vi "Configure923xAcquisition.vi"(8 "error in (no error)":errorcluster) -> (0 "error out":errorcluster, 1 "Register Channel Status Tags":T1[](array[typedef]), 2 "Register Waveform TDMS Properties":T3[](array[typedef]), 3 "923x Acquisition Config":T5={"NumberOfModules"=0, "Dynamic FPGA VI Ref"=refnum, "KeyphasorX3"=[], "FixedSizeX24"={"EnabledChannels"=[], "Sensitivity"=[], "InputConfig"=[]}, "SamplingInfo"={"Number of Channels"=4, "Sampling Rate"=4.0, "Channels"=[], "Units"=[]}, "BlockSize (sec)"=0.0, "Samples To Read (per chan)"=0, "RunningAcquisitionLength"=0.0, "Settling Time"=0.0, "Waveform Groups"=[], "Acquisition Block Number"=0, "Device Name"="", "ValidConfig"=FALSE} {"FixedSizeX24"."InputConfig" items=["AC Coupled", "DC Coupled", "IEPE AC Coupled"]}, 5 "valid":bool)   [LabVIEW 2015]
uses:
  <vilib>/addons/InsightCM/Devices/Shared/AcquireBaseLoop/controls/Configuration.ctl
  <vilib>/addons/InsightCM/Devices/Shared/AcquireBaseLoop/controls/TachometerConfig.ctl
  <vilib>/addons/InsightCM/Devices/Shared/AcquireBaseLoop/controls/FixedSizeArrays.ctl
  <vilib>/LabVIEW Targets/FPGA/cRIO/shared/nicrio_ModuleControls/nicrio_cRIO-9232_ConfigModeRing.ctl
  <vilib>/addons/InsightCM/Devices/Shared/cRIOWfmAcq/subVIs/RIO Wfm Cust Ctrls/rwfm_SamplingInfo.ctl
  <vilib>/addons/InsightCM/Devices/Shared/AcquireBaseLoop/controls/Group.ctl
  <vilib>/addons/InsightCM/Devices/Shared/AcquireBaseLoop/controls/Channel.ctl
  <vilib>/addons/InsightCM/Utilities/ChannelStatus/controls/RangeParams.ctl
  <vilib>/addons/InsightCM/Devices/Shared/TdmsCreator/controls/RegisterWaveformTdmsPropertiesRoutedMessage.ctl
  <vilib>/addons/InsightCM/Devices/Shared/TdmsCreator/controls/Waveform.ctl
  <vilib>/addons/InsightCM/Devices/Shared/TagPublish/controls/PointToPublish.ctl
  <vilib>/addons/PointValueMap/controls/DataTypes.ctl
  <vilib>/addons/InsightCM/Utilities/GlobalConfiguration/GlobalConfiguration.lvlib
  <vilib>/addons/InsightCM/Devices/Shared/AcquireBaseLoop/FpgaAcquisition923x.lvlib
  <vilib>/addons/InsightCM/Devices/Shared/cRIOWfmAcq/cRIOWfmLib.lvlib
  <vilib>/addons/InsightCM/Utilities/ChannelStatus/ChannelStatus.lvlib
  <vilib>/addons/InsightCM/Devices/Shared/TdmsCreator/TdmsCreator.lvlib
  <vilib>/addons/PointValueMap/PointValueMap.lvlib
  <vilib>/addons/InsightCM/Devices/Shared/TagPublish/TagPublish.lvlib
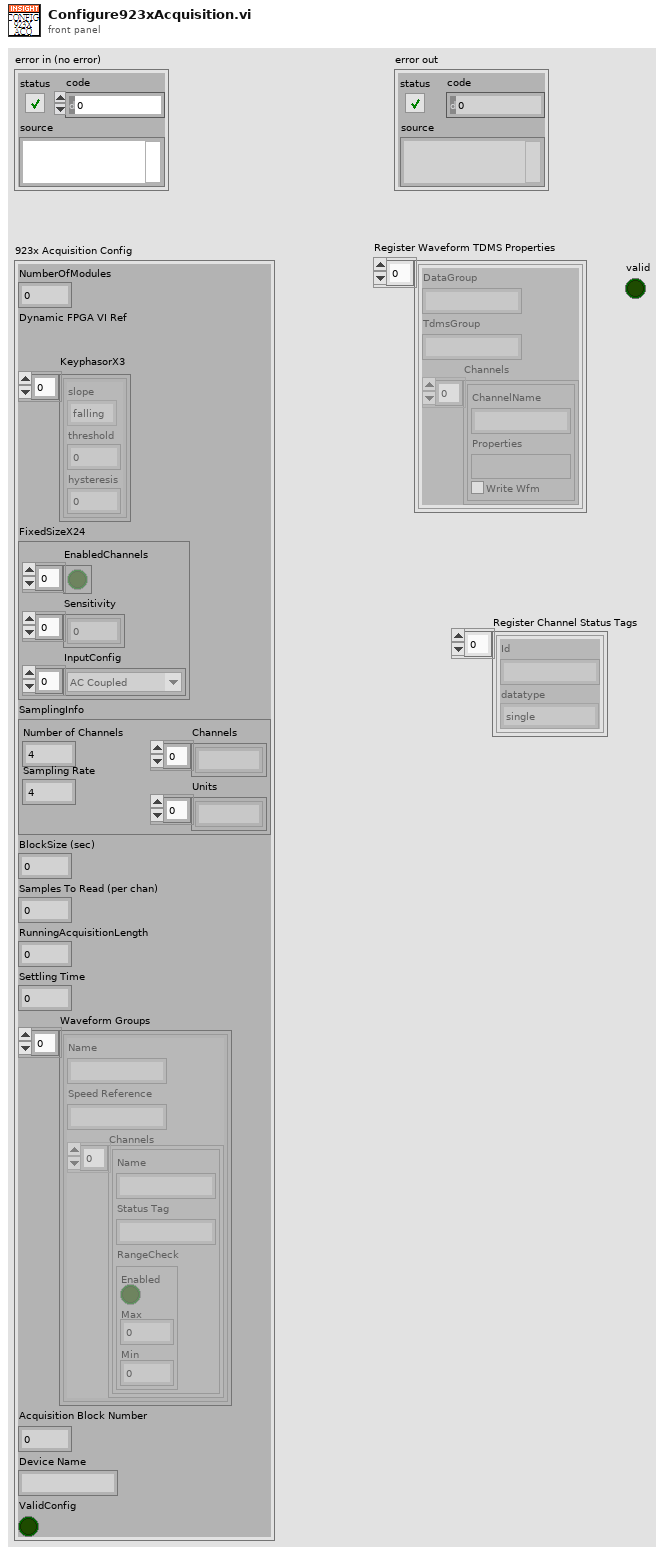
[diagram p1: front panel]
types:
  T1 = typedef "TagPublish.lvlib/PointToPublish.ctl" = cluster{"Id":string, "datatype":T2}
  T2 = typedef "PointValueMap.lvlib/DataTypes.ctl" = enum16{"single", "double", "i32", "string", "variant"}
  T3 = typedef "TdmsCreator.lvlib/RegisterWaveformTdmsPropertiesRoutedMessage.ctl" = cluster{"DataGroup":string, "TdmsGroup":string, "Channels":T4[]}
  T4 = typedef "TdmsCreator.lvlib/Waveform.ctl" = cluster{"ChannelName":string, "Properties":variant, "Write Wfm":bool}
  T5 = typedef "FpgaAcquisition923x.lvlib/Configuration.ctl" = cluster{"NumberOfModules":i16, "Dynamic FPGA VI Ref":refnum<k20>, "KeyphasorX3":T6[], "FixedSizeX24":T7, "SamplingInfo":T9, "BlockSize (sec)":dbl, "Samples To Read (per chan)":i32, "RunningAcquisitionLength":dbl, "Settling Time":dbl, "Waveform Groups":T10[], "Acquisition Block Number":i32, "Device Name":string, "ValidConfig":bool}
  T6 = typedef "FpgaAcquisition923x.lvlib/TachometerConfig.ctl" = cluster{"slope":enum16{"falling", "rising"}, "threshold":dbl, "hysteresis":dbl}
  T7 = typedef "FpgaAcquisition923x.lvlib/FixedSizeArrays.ctl" = cluster{"EnabledChannels":bool[], "Sensitivity":dbl[], "InputConfig":T8[]}
  T8 = typedef "nicrio_cRIO-9232_ConfigModeRing.ctl" = u8
  T9 = typedef "cRIOWfmLib.lvlib/rwfm_SamplingInfo.ctl" = cluster{"Number of Channels":i32, "Sampling Rate":dbl, "Channels":string[], "Units":string[]}
  T10 = typedef "FpgaAcquisition923x.lvlib/Group.ctl" = cluster{"Name":string, "Speed Reference":string, "Channels":T11[]}
  T11 = typedef "FpgaAcquisition923x.lvlib/Channel.ctl" = cluster{"Name":string, "Status Tag":string, "RangeCheck":T12}
  T12 = typedef "ChannelStatus.lvlib/RangeParams.ctl" = cluster{"Enabled":bool, "Max":dbl, "Min":dbl}
  T13 = typedef "Device.ctl" = cluster{"Id":string, "Name":string, "DeviceType":string, "HardwareName":string, "IpAddress":string, "HardwareInfo":T14[], "ApplicationType":string, "ApplicationVersion":string, "EquipmentIds":string[], "ConfigurationVersion":string, "Properties":T14[], "DataGroups":T15[]}
  T14 = typedef "KeyValuePair.ctl" = cluster{"Key":string, "Value":string}
  T15 = typedef "DataGroup.ctl" = cluster{"Name":string, "OperatingStates":T16[], "Properties":T14[], "EquipmentIds":string[]}
  T16 = typedef "OperatingState.ctl" = cluster{"Name":string, "Properties":T14[], "Triggers":T17[]}
  T17 = typedef "Trigger.ctl" = cluster{"Type":string, "Expression":string, "Conditions":T18[]}
  T18 = typedef "Condition.ctl" = cluster{"Source":string, "Type":string, "Operator":string, "CompareTo":string, "DwellSeconds":dbl}
  T19 = typedef "Channel.ctl" = cluster{"Id":string, "DeviceId":string, "Name":string, "ChannelType":string, "HardwareKey":string, "HardwareChannel":string, "DataGroup":string, "Keywords":string[], "EquipmentIds":string[], "Properties":T14[], "Metrics":T20[]}
  T20 = typedef "MetricModel.ctl" = cluster{"Id":string, "MetricDefinitionInstanceId":string, "Properties":T14[]}
  T21 = typedef "Equipment.ctl" = cluster{"Id":string, "ParentId":string, "Levelname":string, "Name":string, "Properties":T14[]}
  T22 = typedef "Tag.ctl" = cluster{"Id":string, "Path":string, "Name":string, "Datatype":string, "Props":T14[], "Keywords":string[]}
  T23 = typedef "SectionKeyValues.ctl" = cluster{"Section":string, "KeyValues":T14[]}
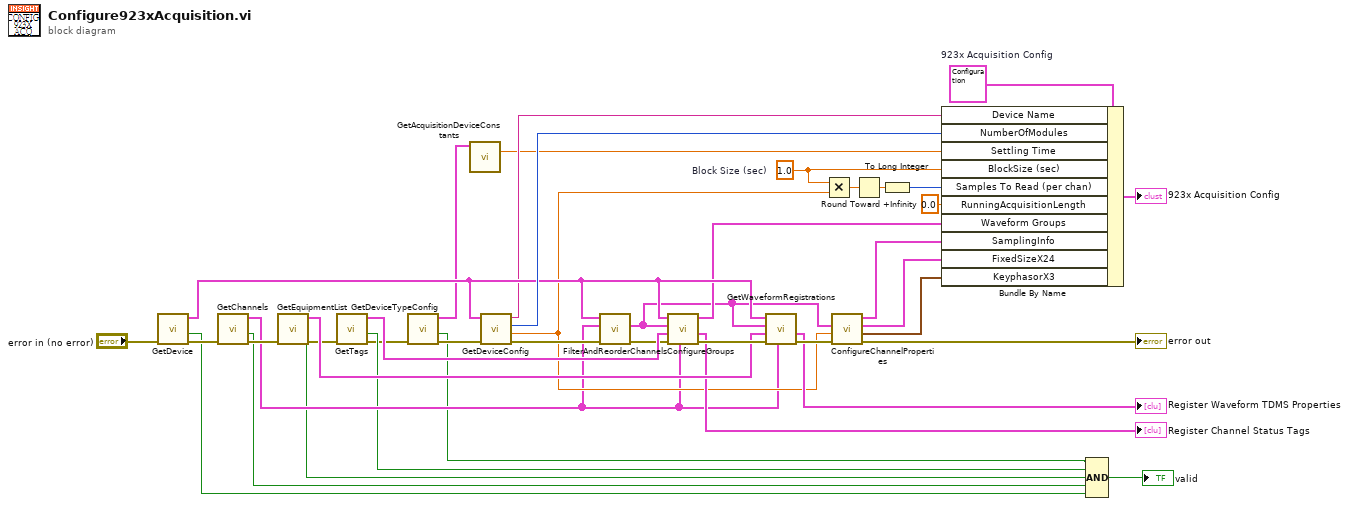
[diagram p0: block diagram]
diagram:
  w29 = T5 {"NumberOfModules"=0, "Dynamic FPGA VI Ref"=refnum, "KeyphasorX3"=[], "FixedSizeX24"={"EnabledChannels"=[], "Sensitivity"=[], "InputConfig"=[]}, "SamplingInfo"={"Number of Channels"=4, "Sampling Rate"=4.0, "Channels"=[], "Units"=[]}, "BlockSize (sec)"=0.0, "Samples To Read (per chan)"=0, "RunningAcquisitionLength"=0.0, "Settling Time"=0.0, "Waveform Groups"=[], "Acquisition Block Number"=0, "Device Name"="", "ValidConfig"=FALSE}  # 923x Acquisition Config
  w36 = 1.0  # Block Size (sec)
  n1 = call <vilib>:"GetDevice.vi"("error in (no error)"="error in (no error)") -> ("error out"=w39:errorcluster, "found"=w10:bool, "device configuration"=w22:T13)  [unwired: 8 in]
  n2 = call <vilib>:"GetChannels.vi"("error in (no error)"=w39) -> ("error out"=w20:errorcluster, "found"=w9:bool, "channels"=w11:T19[])  [unwired: 8 in]
  n3 = call <vilib>:"GetEquipmentList.vi"("error in (no error)"=w20) -> ("error out"=w19:errorcluster, "found"=w8:bool, "equipment list"=w21:T21[])  [unwired: 8 in]
  n4 = call <vilib>:"GetTags.vi"("error in (no error)"=w19) -> ("error out"=w5:errorcluster, "found"=w7:bool, "tags"=w26:T22[])  [unwired: 8 in]
  n5 = call <vilib>:"GetDeviceTypeConfig.vi"("error in (no error)"=w5) -> ("error out"=w4:errorcluster, "found"=w1:bool, "key values"=w3:T23[])  [unwired: 8 in]
  n6 = call <vilib>:"GetAcquisitionDeviceConstants.vi"("key values"=w3) -> ("settling time (seconds)"=w2:dbl)  [unwired: 10 in]
  n7 = call <vilib>:"GetDeviceConfig.vi"("error in (no error)"=w4, "Device"=w22) -> ("error out"=w28:errorcluster, "Sample Rate"=w13:dbl, "Number of Dynamic Modules"=w33:i32, "Name"=w16:string)  [unwired: 6 in]
  n8 = call "FilterAndReorderChannels.vi"("error in (no error)"=w28, "channels"=w11, "device"=w22) -> ("error out"=w25:errorcluster, "acquisition channels (in acquisition order)"=w12:T19[])  [unwired: 7 in]
  n9 = call <vilib>:"ConfigureGroups.vi"("all channels"=w11, "error in (no error)"=w25, "tags"=w26, "acquisition channels (in acquisition order)"=w12, "device"=w22) -> ("error out"=w24:errorcluster, "register channel status tags"=→"Register Channel Status Tags":T1[], "groups"=w17:T10[])  [unwired: 4 in]
  n10 = call <vilib>:"GetWaveformRegistrations.vi"("all channels"=w11, "error in (no error)"=w24, "equipment list"=w21, "acquisition channels (in acquisition order)"=w12, "device"=w22) -> ("error out"=w23:errorcluster, "register waveform tdms properties"=→"Register Waveform TDMS Properties":T3[])  [unwired: 5 in]
  n11 = Multiply(x=w36, y=w13) -> (x*y=w38:dbl)
  n12 = call <vilib>:"ConfigureChannelProperties.vi"("error in (no error)"=w23, "Sampling Rate"=w13, "Filtered Channels (in acquisition order)"=w12) -> ("error out"=→"error out":errorcluster, "Tach Config X3"=w31:T6[], "Channel Config X24"=w32:T7, "Sampling Info"=w18:T9)  [unwired: 5 in]
  n13 = Round Toward +Infinity(x=w38) -> (ceil(x): smallest int >= x=w37:dbl)
  n14 = To Long Integer(number=w37) -> (32bit integer=w35:i32)
  n15 = Bundle By Name(cluster=w29, "Device Name"=w16, "NumberOfModules"=w33, "Settling Time"=w2, "BlockSize (sec)"=w36, "Samples To Read (per chan)"=w35, "RunningAcquisitionLength"=0.0, "Waveform Groups"=w17, "SamplingInfo"=w18, "FixedSizeX24"=w32, "KeyphasorX3"=w31) -> (→"923x Acquisition Config":T5)
  n16 = Compound Arithmetic op=AND(w1, w7, w8, w9, w10) -> (→"valid":bool)
